vi "CCalAmounts_main.vi"() -> ()   [LabVIEW 2013]
uses:
  Instance           5 24Saved   CCalAmounts_main .vi
panel:
  in  "export type":u16(ring) items=["measure script", "masslynx"]
  in  "export to clipboard button":bool
  in  "exit button":bool
  in  "export to file button":bool
  in  "save button":bool
  in  "load button":bool
  in  "error in (no error)":errorcluster
  in  "additional vol. [ml]":dbl=11.0
  in  "pipette vol. [ml]":dbl=0.2148
  out "amount of istopes":i32(listbox)
  out "mols in Cal-volume":dbl format="%#.6g"
  in  "calibration vol. [ml]":dbl=10670.0
  out "dry pressure [mbar]":dbl format="%#.6g"
  out "water.vap.press [mbar]":dbl format="%#.6g"
  in  "humidity [%]":dbl
  in  "temperature [°C]":dbl=21.0
  in  "pressure [mbar]":dbl=990.0
  in  "Standard name":string
  # "standard amounts for air standards"
  # "Standard Conditions:"
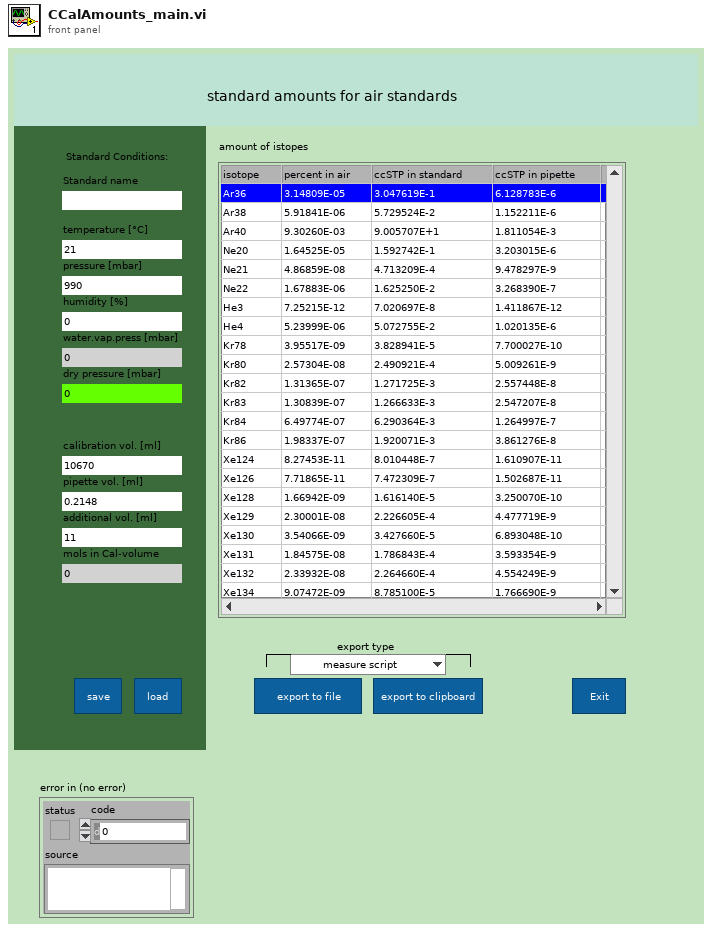
[diagram p1: front panel]
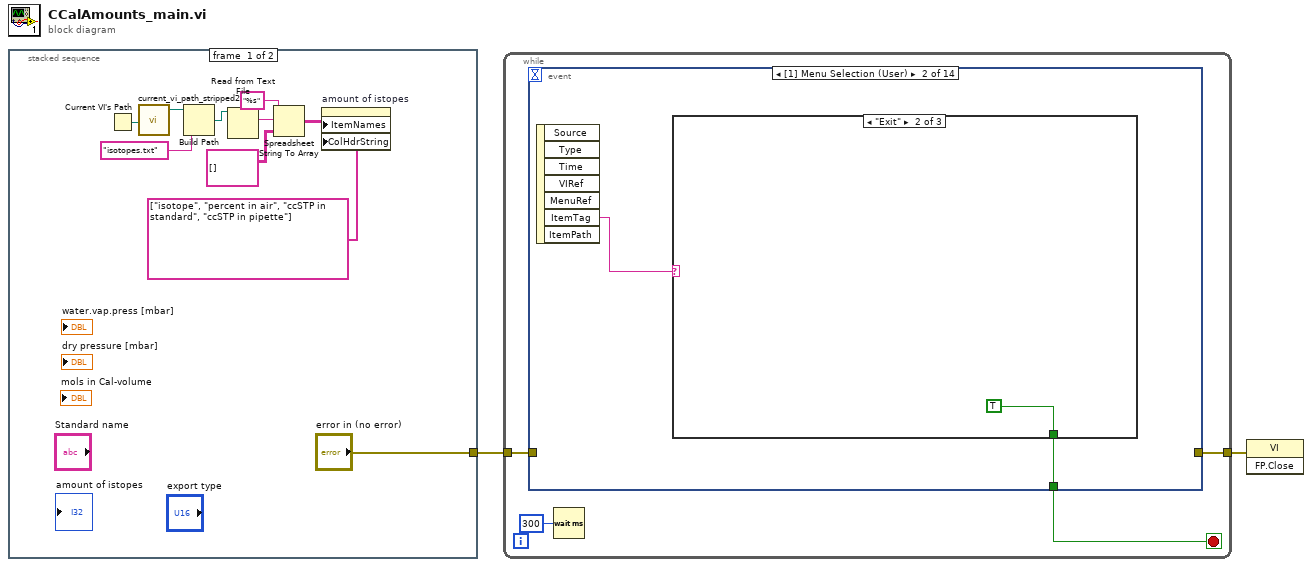
[diagram p0: block diagram]
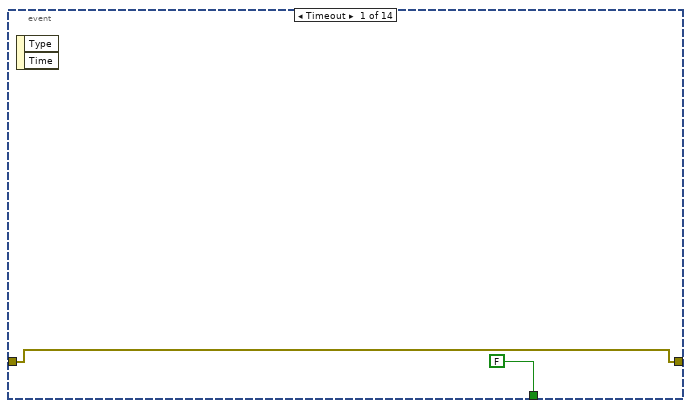
[diagram p2: hidden frame]
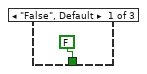
[diagram p3: hidden frame]
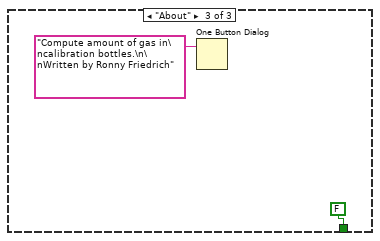
[diagram p4: hidden frame]
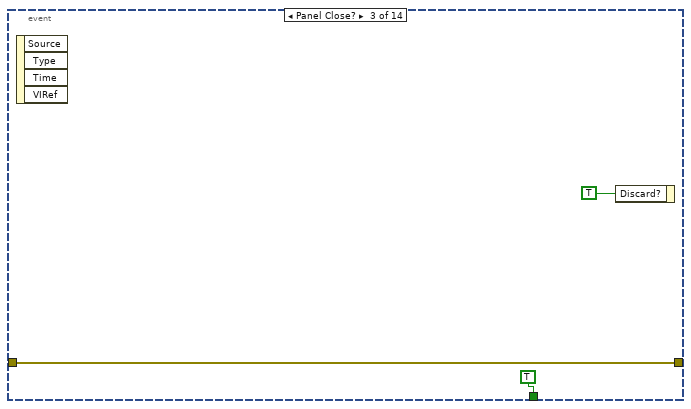
[diagram p5: hidden frame]
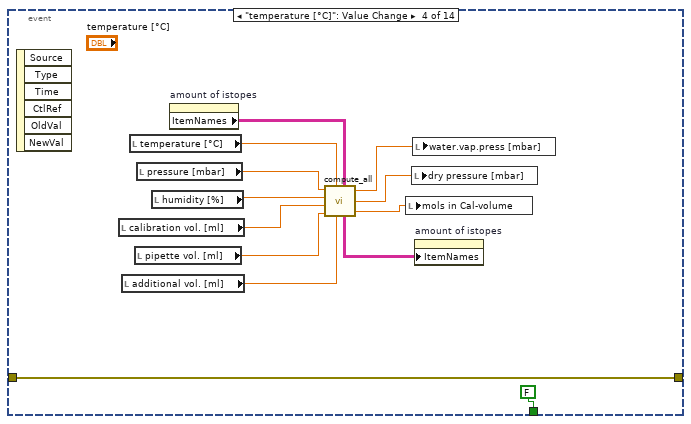
[diagram p6: hidden frame]
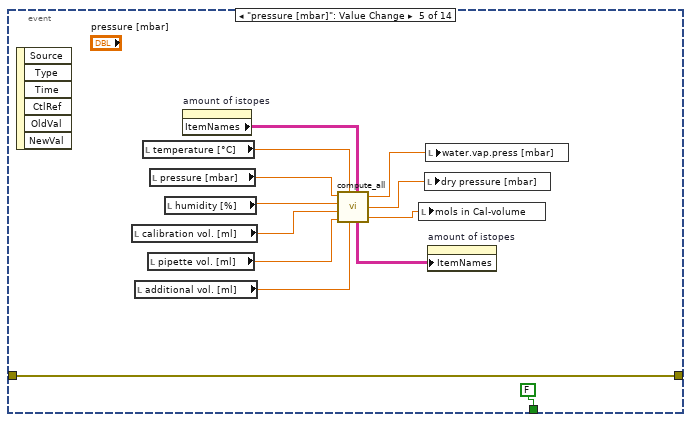
[diagram p7: hidden frame]
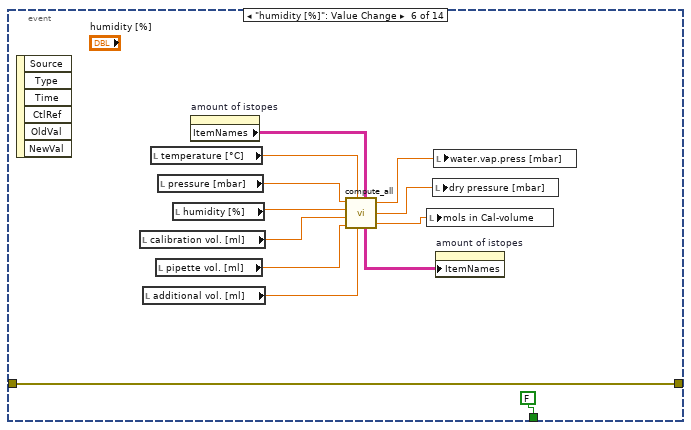
[diagram p8: hidden frame]
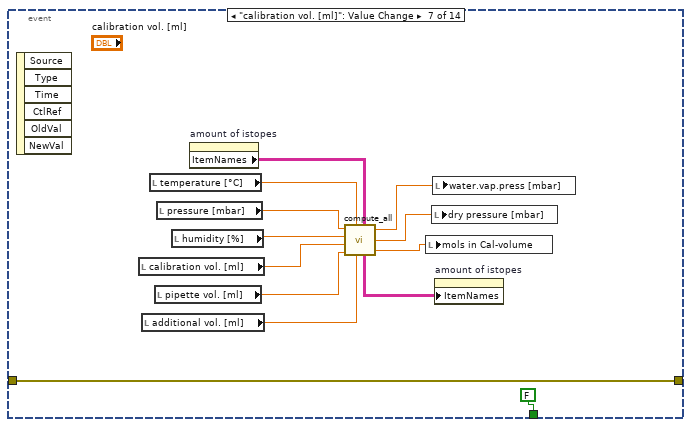
[diagram p9: hidden frame]
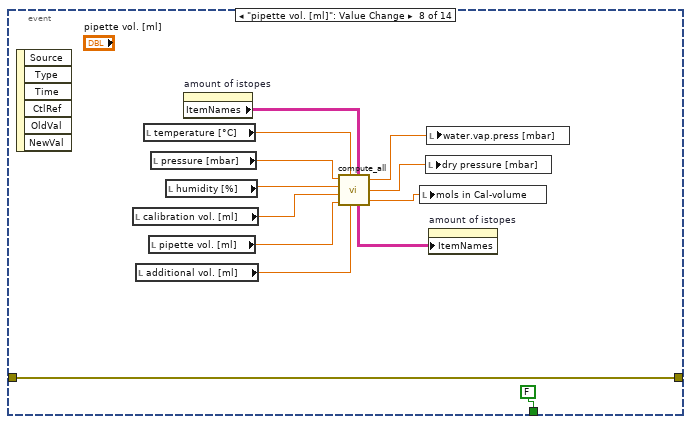
[diagram p10: hidden frame]
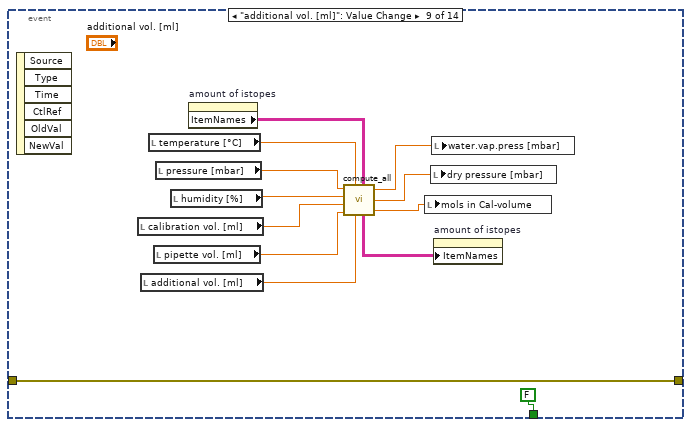
[diagram p11: hidden frame]
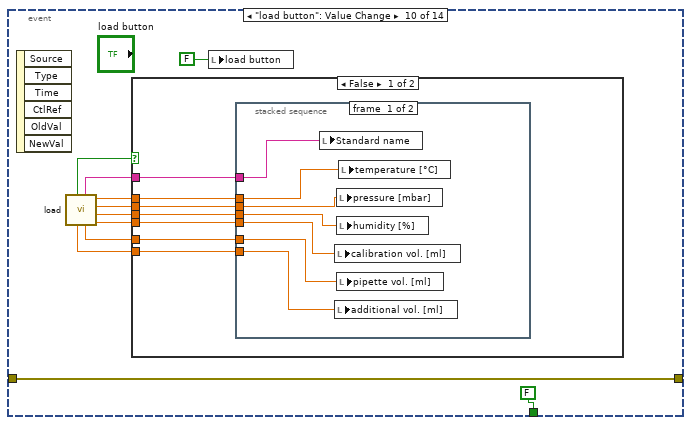
[diagram p12: hidden frame]
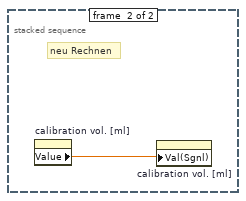
[diagram p13: hidden frame]
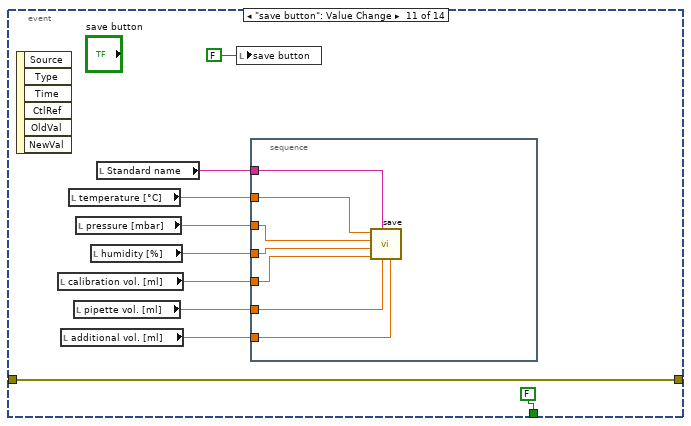
[diagram p15: hidden frame]
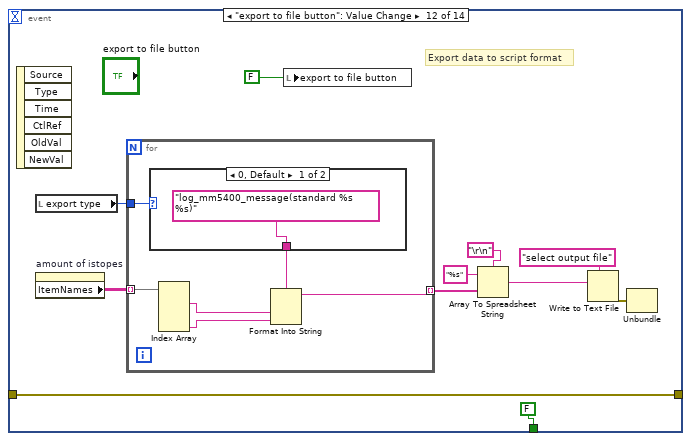
[diagram p16: hidden frame]
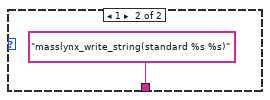
[diagram p17: hidden frame]
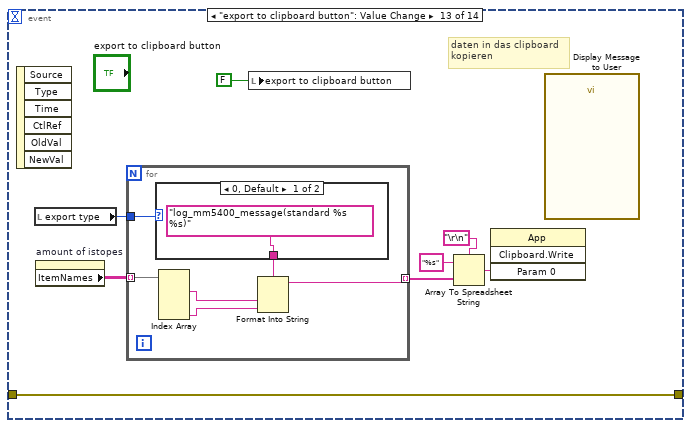
[diagram p18: hidden frame]
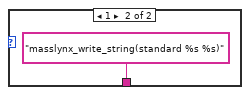
[diagram p19: hidden frame]
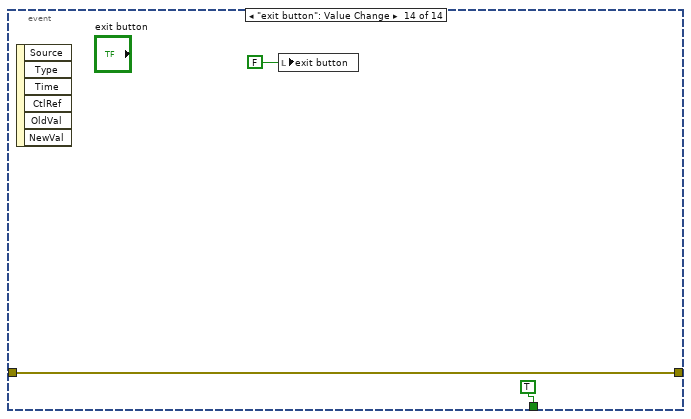
[diagram p20: hidden frame]
diagram:
  n1 = stacked-sequence {
    tunnel: ["error in (no error)" _] -> w2
    frame #0 {
      n2 = Current VI's Path() -> (path=w12:path)
      n3 = call "current_vi_path_stripped2.vi"("current VI Path"=w12) -> ("current VI Path stripped out"=w11:path)  [unwired: 3 in, 1 out]
      n4 = Build Path(base path=w11, name or relative path="isotopes.txt") -> (appended path=w9:path)
      n5 = Read from Text File(file (use dialog)=w9) -> (text=w8:string)  [unwired: 3 in, 3 out]
      n6 = Spreadsheet String To Array(format string="%s", spreadsheet string=w8, array type (2D Dbl)=string[][] []) -> (array=w5:string[][])  [unwired: 1 in]
      n7 = property on="amount of istopes" class="MCListbox (strict)"("ItemNames"=w5, "ColHdrString"=string[] ["isotope", "percent in air", "ccSTP in standard", "ccSTP in pipette"] ("Column Header Strings[]")) -> ()  [unwired: 2 in, 2 out]
    }
    frame #1 {
      # "calculate everything for known values"
      n8 = local read "calibration vol. [ml]"() -> (w17:dbl)
      n9 = local read "additional vol. [ml]"() -> (w19:dbl)
      n10 = local read "temperature [°C]"() -> (w14:dbl)
      n11 = local read "pipette vol. [ml]"() -> (w18:dbl)
      n12 = local read "pressure [mbar]"() -> (w15:dbl)
      n13 = local read "humidity [%]"() -> (w16:dbl)
      n14 = property on="amount of istopes" class="MCListbox (strict)"() -> ("ItemNames"=w13:string[][])  [unwired: 2 in, 2 out]
      n15 = call "compute_all.vi"("ItemNames"=w13, "additional vol. [ml]"=w19, "pipette vol. [ml]"=w18, "calibration vol. [ml]"=w17, "temperature [°C]"=w14, "humidity [%]"=w16, "pressure [mbar]"=w15) -> ("mols"=w22:dbl, "Array"=w23:string[][], "pout"=w21:dbl, "wvp"=w20:dbl)
      n16 = local write "mols in Cal-volume"(w22) -> ()
      n17 = local write "dry pressure [mbar]"(w21) -> ()
      n18 = local write "water.vap.press [mbar]"(w20) -> ()
      n19 = property on="amount of istopes" class="MCListbox (strict)"("ItemNames"=w23) -> ()  [unwired: 2 in, 2 out]
    }
  }
  n20 = while {
    tunnel: w2 -> [w25]
    tunnel: [w24] -> w1
    stop <- w26 stop-if-true
    n21 = event shown="[1] Menu Selection (User)" {
      selector: _ -> [_ _ _ _ _ _ _ _ _ _ _ _ _ _]
      dyn-events: _ -> [_ _ _ _ _ _ _ _ _ _ _ _ _ _]
      timeout: _ -> [_ _ _ _ _ _ _ _ _ _ _ _ _ _]
      tunnel: [FALSE w30 TRUE FALSE FALSE FALSE FALSE FALSE FALSE FALSE FALSE FALSE _ TRUE] -> w26
      tunnel: w25 -> [w28 _ w36 w39 w52 w65 w78 w91 w104 w117 w143 w161 w180 w195]
      tunnel: [w28 _ w36 w39 w52 w65 w78 w91 w104 w117 w143 w161 w180 w195] -> w24
      event Timeout {
        n22 = event-data() -> ()  [unwired: 1 in, 2 out]
      }
      event Menu Selection (User) {
        n23 = event-data() -> ("ItemTag"=w31:string)  [unwired: 1 in, 6 out]
        n24 = case shown="\"Exit\"" w31 {
          tunnel: [FALSE TRUE FALSE] -> w30
          frame "False", Default {
          }
          frame "Exit" {
          }
          frame "About" {
            n25 = One Button Dialog(message="Compute amount of gas in\ncalibration bottles.\n\nWritten by Ronny Friedrich") -> ()  [unwired: 1 in, 1 out]
          }
        }
      }
      event Panel Close? {
        n26 = event-data() -> ()  [unwired: 1 in, 4 out]
        n27 = event-data("Discard?"=TRUE) -> ()  [unwired: 1 in, 1 out]
      }
      event "temperature [°C]": Value Change {
        n28 = event-data() -> ()  [unwired: 1 in, 6 out]
        n29 = local read "calibration vol. [ml]"() -> (w45:dbl)
        n30 = local read "additional vol. [ml]"() -> (w47:dbl)
        n31 = local read "temperature [°C]"() -> (w42:dbl)
        n32 = local read "pipette vol. [ml]"() -> (w46:dbl)
        n33 = local read "pressure [mbar]"() -> (w43:dbl)
        n34 = local read "humidity [%]"() -> (w44:dbl)
        n35 = property on="amount of istopes" class="MCListbox (strict)"() -> ("ItemNames"=w41:string[][])  [unwired: 2 in, 2 out]
        n36 = call "compute_all.vi"("ItemNames"=w41, "additional vol. [ml]"=w47, "pipette vol. [ml]"=w46, "calibration vol. [ml]"=w45, "temperature [°C]"=w42, "humidity [%]"=w44, "pressure [mbar]"=w43) -> ("mols"=w50:dbl, "Array"=w51:string[][], "pout"=w49:dbl, "wvp"=w48:dbl)
        n37 = local write "mols in Cal-volume"(w50) -> ()
        n38 = local write "dry pressure [mbar]"(w49) -> ()
        n39 = local write "water.vap.press [mbar]"(w48) -> ()
        n40 = property on="amount of istopes" class="MCListbox (strict)"("ItemNames"=w51) -> ()  [unwired: 2 in, 2 out]
      }
      event "pressure [mbar]": Value Change {
        n41 = event-data() -> ()  [unwired: 1 in, 6 out]
        n42 = local read "calibration vol. [ml]"() -> (w58:dbl)
        n43 = local read "additional vol. [ml]"() -> (w60:dbl)
        n44 = local read "temperature [°C]"() -> (w55:dbl)
        n45 = local read "pipette vol. [ml]"() -> (w59:dbl)
        n46 = local read "pressure [mbar]"() -> (w56:dbl)
        n47 = local read "humidity [%]"() -> (w57:dbl)
        n48 = property on="amount of istopes" class="MCListbox (strict)"() -> ("ItemNames"=w54:string[][])  [unwired: 2 in, 2 out]
        n49 = call "compute_all.vi"("ItemNames"=w54, "additional vol. [ml]"=w60, "pipette vol. [ml]"=w59, "calibration vol. [ml]"=w58, "temperature [°C]"=w55, "humidity [%]"=w57, "pressure [mbar]"=w56) -> ("mols"=w63:dbl, "Array"=w64:string[][], "pout"=w62:dbl, "wvp"=w61:dbl)
        n50 = local write "mols in Cal-volume"(w63) -> ()
        n51 = local write "dry pressure [mbar]"(w62) -> ()
        n52 = local write "water.vap.press [mbar]"(w61) -> ()
        n53 = property on="amount of istopes" class="MCListbox (strict)"("ItemNames"=w64) -> ()  [unwired: 2 in, 2 out]
      }
      event "humidity [%]": Value Change {
        n54 = event-data() -> ()  [unwired: 1 in, 6 out]
        n55 = local read "calibration vol. [ml]"() -> (w71:dbl)
        n56 = local read "additional vol. [ml]"() -> (w73:dbl)
        n57 = local read "temperature [°C]"() -> (w68:dbl)
        n58 = local read "pipette vol. [ml]"() -> (w72:dbl)
        n59 = local read "pressure [mbar]"() -> (w69:dbl)
        n60 = local read "humidity [%]"() -> (w70:dbl)
        n61 = property on="amount of istopes" class="MCListbox (strict)"() -> ("ItemNames"=w67:string[][])  [unwired: 2 in, 2 out]
        n62 = call "compute_all.vi"("ItemNames"=w67, "additional vol. [ml]"=w73, "pipette vol. [ml]"=w72, "calibration vol. [ml]"=w71, "temperature [°C]"=w68, "humidity [%]"=w70, "pressure [mbar]"=w69) -> ("mols"=w76:dbl, "Array"=w77:string[][], "pout"=w75:dbl, "wvp"=w74:dbl)
        n63 = local write "mols in Cal-volume"(w76) -> ()
        n64 = local write "dry pressure [mbar]"(w75) -> ()
        n65 = local write "water.vap.press [mbar]"(w74) -> ()
        n66 = property on="amount of istopes" class="MCListbox (strict)"("ItemNames"=w77) -> ()  [unwired: 2 in, 2 out]
      }
      event "calibration vol. [ml]": Value Change {
        n67 = event-data() -> ()  [unwired: 1 in, 6 out]
        n68 = local read "calibration vol. [ml]"() -> (w84:dbl)
        n69 = local read "additional vol. [ml]"() -> (w86:dbl)
        n70 = local read "temperature [°C]"() -> (w81:dbl)
        n71 = local read "pipette vol. [ml]"() -> (w85:dbl)
        n72 = local read "pressure [mbar]"() -> (w82:dbl)
        n73 = local read "humidity [%]"() -> (w83:dbl)
        n74 = property on="amount of istopes" class="MCListbox (strict)"() -> ("ItemNames"=w80:string[][])  [unwired: 2 in, 2 out]
        n75 = call "compute_all.vi"("ItemNames"=w80, "additional vol. [ml]"=w86, "pipette vol. [ml]"=w85, "calibration vol. [ml]"=w84, "temperature [°C]"=w81, "humidity [%]"=w83, "pressure [mbar]"=w82) -> ("mols"=w89:dbl, "Array"=w90:string[][], "pout"=w88:dbl, "wvp"=w87:dbl)
        n76 = local write "mols in Cal-volume"(w89) -> ()
        n77 = local write "dry pressure [mbar]"(w88) -> ()
        n78 = local write "water.vap.press [mbar]"(w87) -> ()
        n79 = property on="amount of istopes" class="MCListbox (strict)"("ItemNames"=w90) -> ()  [unwired: 2 in, 2 out]
      }
      event "pipette vol. [ml]": Value Change {
        n80 = event-data() -> ()  [unwired: 1 in, 6 out]
        n81 = local read "calibration vol. [ml]"() -> (w97:dbl)
        n82 = local read "additional vol. [ml]"() -> (w99:dbl)
        n83 = local read "temperature [°C]"() -> (w94:dbl)
        n84 = local read "pipette vol. [ml]"() -> (w98:dbl)
        n85 = local read "pressure [mbar]"() -> (w95:dbl)
        n86 = local read "humidity [%]"() -> (w96:dbl)
        n87 = property on="amount of istopes" class="MCListbox (strict)"() -> ("ItemNames"=w93:string[][])  [unwired: 2 in, 2 out]
        n88 = call "compute_all.vi"("ItemNames"=w93, "additional vol. [ml]"=w99, "pipette vol. [ml]"=w98, "calibration vol. [ml]"=w97, "temperature [°C]"=w94, "humidity [%]"=w96, "pressure [mbar]"=w95) -> ("mols"=w102:dbl, "Array"=w103:string[][], "pout"=w101:dbl, "wvp"=w100:dbl)
        n89 = local write "mols in Cal-volume"(w102) -> ()
        n90 = local write "dry pressure [mbar]"(w101) -> ()
        n91 = local write "water.vap.press [mbar]"(w100) -> ()
        n92 = property on="amount of istopes" class="MCListbox (strict)"("ItemNames"=w103) -> ()  [unwired: 2 in, 2 out]
      }
      event "additional vol. [ml]": Value Change {
        n93 = event-data() -> ()  [unwired: 1 in, 6 out]
        n94 = local read "calibration vol. [ml]"() -> (w110:dbl)
        n95 = local read "additional vol. [ml]"() -> (w112:dbl)
        n96 = local read "temperature [°C]"() -> (w107:dbl)
        n97 = local read "pipette vol. [ml]"() -> (w111:dbl)
        n98 = local read "pressure [mbar]"() -> (w108:dbl)
        n99 = local read "humidity [%]"() -> (w109:dbl)
        n100 = property on="amount of istopes" class="MCListbox (strict)"() -> ("ItemNames"=w106:string[][])  [unwired: 2 in, 2 out]
        n101 = call "compute_all.vi"("ItemNames"=w106, "additional vol. [ml]"=w112, "pipette vol. [ml]"=w111, "calibration vol. [ml]"=w110, "temperature [°C]"=w107, "humidity [%]"=w109, "pressure [mbar]"=w108) -> ("mols"=w115:dbl, "Array"=w116:string[][], "pout"=w114:dbl, "wvp"=w113:dbl)
        n102 = local write "mols in Cal-volume"(w115) -> ()
        n103 = local write "dry pressure [mbar]"(w114) -> ()
        n104 = local write "water.vap.press [mbar]"(w113) -> ()
        n105 = property on="amount of istopes" class="MCListbox (strict)"("ItemNames"=w116) -> ()  [unwired: 2 in, 2 out]
      }
      event "load button": Value Change {
        n106 = event-data() -> ()  [unwired: 1 in, 6 out]
        n107 = call "load.vi"() -> ("calibration vol. [ml]"=w120:dbl, "humidity [%]"=w121:dbl, "pressure [mbar]"=w122:dbl, "temperature [°C]"=w123:dbl, "pipette vol. [ml]"=w119:dbl, "CA-Name"=w124:string, "additional vol. [ml]"=w118:dbl, "canceled?"=w125:bool)  [unwired: 4 in]
        n108 = case shown="False" w125 {
          tunnel: w124 -> [w134 _]
          tunnel: w123 -> [w133 _]
          tunnel: w122 -> [w132 _]
          tunnel: w121 -> [w131 _]
          tunnel: w120 -> [w130 _]
          tunnel: w119 -> [w129 _]
          tunnel: w118 -> [w128 _]
          frame False {
            n109 = stacked-sequence {
              tunnel: w134 -> [w141 _]
              tunnel: w133 -> [w140 _]
              tunnel: w132 -> [w139 _]
              tunnel: w131 -> [w138 _]
              tunnel: w130 -> [w137 _]
              tunnel: w129 -> [w136 _]
              tunnel: w128 -> [w135 _]
              frame #0 {
                n110 = local write "Standard name"(w141) -> ()
                n111 = local write "calibration vol. [ml]"(w137) -> ()
                n112 = local write "additional vol. [ml]"(w135) -> ()
                n113 = local write "pressure [mbar]"(w139) -> ()
                n114 = local write "humidity [%]"(w138) -> ()
                n115 = local write "pipette vol. [ml]"(w136) -> ()
                n116 = local write "temperature [°C]"(w140) -> ()
              }
              frame #1 {
                # "neu Rechnen"
                n117 = property on="calibration vol. [ml]" class="DigNum (strict)"() -> ("Value"=w142:dbl)  [unwired: 2 in, 2 out]
                n118 = property on="calibration vol. [ml]" class="DigNum (strict)"("Val(Sgnl)"=w142) -> ()  [unwired: 2 in, 2 out]
              }
            }
          }
          frame True {
            # "es wurde nichts geladen"
          }
        }
        n119 = local write "load button"(FALSE ("load button")) -> ()
      }
      event "save button": Value Change {
        n120 = event-data() -> ()  [unwired: 1 in, 6 out]
        n121 = local read "calibration vol. [ml]"() -> (w148:dbl)
        n122 = local read "additional vol. [ml]"() -> (w150:dbl)
        n123 = local read "temperature [°C]"() -> (w145:dbl)
        n124 = local read "pipette vol. [ml]"() -> (w149:dbl)
        n125 = local read "pressure [mbar]"() -> (w146:dbl)
        n126 = local read "humidity [%]"() -> (w147:dbl)
        n127 = local read "Standard name"() -> (w144:string)
        n128 = local write "save button"(FALSE ("save button")) -> ()
        n129 = stacked-sequence {
          tunnel: w150 -> [w153]
          tunnel: w149 -> [w154]
          tunnel: w148 -> [w155]
          tunnel: w147 -> [w156]
          tunnel: w146 -> [w157]
          tunnel: w145 -> [w158]
          tunnel: w144 -> [w159]
          frame #0 {
            n130 = call "save.vi"("additional vol. [ml]"=w153, "pipette vol. [ml]"=w154, "CA-Name"=w159, "calibration vol. [ml]"=w155, "humidity [%]"=w156, "pressure [mbar]"=w157, "temperature [°C]"=w158) -> ()  [unwired: 5 in]
          }
        }
      }
      event "export to file button": Value Change {
        # "Export data to script format"
        n131 = event-data() -> ()  [unwired: 1 in, 6 out]
        n132 = local read "export type"() -> (w160:u16)
        n133 = property on="amount of istopes" class="MCListbox (strict)"() -> ("ItemNames"=w168:string[][])  [unwired: 2 in, 2 out]
        n134 = for {
          tunnel: w168 -> [w176] mode=indexing
          tunnel: [w172] -> w167 mode=indexing
          tunnel: w160 -> [w171]
          n135 = case shown="0, Default" w171 {
            tunnel: ["log_mm5400_message(standard %s %s)" ("format string") "masslynx_write_string(standard %s %s)" ("format string")] -> w175
            frame 0, Default {
            }
            frame 1 {
            }
          }
          n136 = Index Array(array=w176) -> (element #1=w174:string, element #4=w173:string)  [unwired: 4 in, 2 out]
          n137 = Format Into String(format string=w175, w174, w173) -> (resulting string=w172:string)  [unwired: 2 in, 1 out]
        }
        n138 = local write "export to file button"(FALSE ("export button")) -> ()
        n139 = Array To Spreadsheet String(delimiter (Tab)="\r\n", array=w167, 3:"%s" ("format string")) -> (spreadsheet string=w164:string)
        n140 = Write to Text File(prompt (Choose or enter file path)="select output file", text=w164) -> (error out=w163:errorcluster)  [unwired: 2 in, 2 out]
        n141 = Unbundle(w163) -> ()  [unwired: 3 out]
      }
      event "export to clipboard button": Value Change {
        # "daten in das clipboard\nkopieren"
        n142 = event-data() -> ()  [unwired: 1 in, 6 out]
        n143 = local read "export type"() -> (w179:u16)
        n144 = property on="amount of istopes" class="MCListbox (strict)"() -> ("ItemNames"=w185:string[][])  [unwired: 2 in, 2 out]
        n145 = for {
          tunnel: w185 -> [w192] mode=indexing
          tunnel: [w189] -> w184 mode=indexing
          tunnel: w179 -> [w187]
          n146 = case shown="0, Default" w187 {
            tunnel: ["log_mm5400_message(standard %s %s)" ("format string") "masslynx_write_string(standard %s %s)" ("format string")] -> w188
            frame 0, Default {
            }
            frame 1 {
            }
          }
          n147 = Index Array(array=w192) -> (element #1=w191:string, element #4=w190:string)  [unwired: 4 in, 2 out]
          n148 = Format Into String(format string=w188, w191, w190) -> (resulting string=w189:string)  [unwired: 2 in, 1 out]
        }
        n149 = local write "export to clipboard button"(FALSE ("export to clipboard button")) -> ()
        n150 = Array To Spreadsheet String(delimiter (Tab)="\r\n", array=w184, 3:"%s" ("format string")) -> (spreadsheet string=w181:string)
        n151 = invoke class="App" method="Clipboard.Write"("Param 0"=w181) -> ()  [unwired: 3 in, 4 out]
        n152 = call "Display Message to User"() -> ()  [unwired: 10 in, 2 out]
      }
      event "exit button": Value Change {
        n153 = event-data() -> ()  [unwired: 1 in, 6 out]
        n154 = local write "exit button"(FALSE ("exit button")) -> ()
      }
    }
    n155 = Wait (ms)(milliseconds to wait=u32 300) -> ()  [unwired: 1 out]
  }
  n156 = invoke class="VI" method="FP.Close"(error in=w1) -> ()  [unwired: 2 in, 3 out]
